vi "LVDimInterface.dic_command_service_local.vi"(1 "commandID":i32, 3 "data":string, 5 "error in (no error)":errorcluster) -> (15 "success":i32, 19 "error out":errorcluster)   [LabVIEW 2015, in "LVDimInterface.lvlib"]
doc: "This routine requests the execution of a command on the local (THIS) server, address and size contain the command parameters.\n\nThis routine allows clients (user interfaces for ex.) to send commands to be executed by internal servers.\n\nHistory: 16-DEC-2005, Dietrich Beck\n\nCopyright (C)\nGesellschaft für Schwerionenforschung, GSI\nPlanckstr. 1\n64291 Darmstadt\nGermany\n\nContact: D.Beck@gsi.de \n\nThis program is free software; you can redistribute it and/or modify it under the terms of the \nGNU General Public License as published by the Free Software Foundation; either version 2 of the license, or (at your option) any later version.\n\nThis program is distributed in the hope that it will be useful, but WITHOUT ANY WARRANTY; without even the implied warranty of MERCHANTABILITY or FITNESS FOR A PARTICULAR PURPOSE. See the GNU General License for more details (http://www.gnu.org).\n\nGesellschaft für Schwerionenforschung, GSI\nPlanckstr. 1, 64291 Darmstadt, Germany\nFor all questions and ideas contact D. Beck.\nLast update: 16-DEC-2005"
uses:
  LVDimInterface.lvlib
  LVDimInterface.queue type.ctl
  LVDimInterface.notifier type.ctl
panel:
  in  "notifierRef":T1
  in  "queueRef":T2
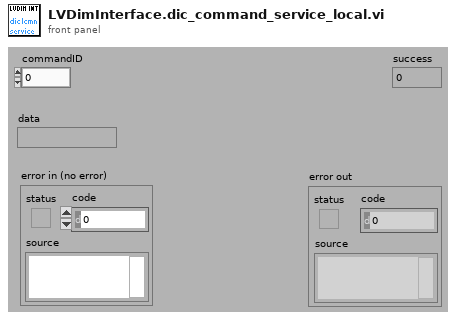
[diagram p1: front panel]
types:
  T1 = typedef "LVDimInterface.lvlib/LVDimInterface.notifier type.ctl" = refnum<notifier>
  T2 = typedef "LVDimInterface.lvlib/LVDimInterface.queue type.ctl" = refnum<queue>
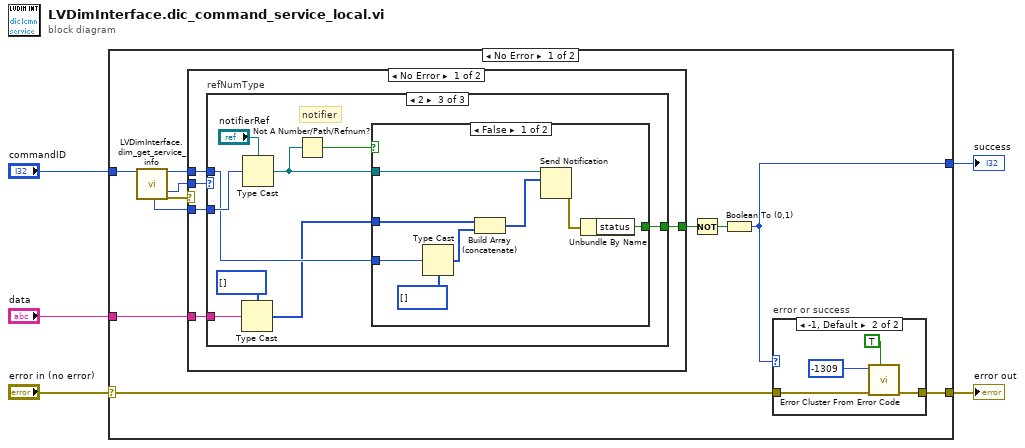
[diagram p0: block diagram]
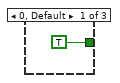
[diagram p2: hidden frame]
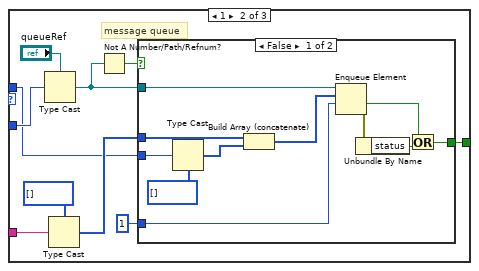
[diagram p3: hidden frame]
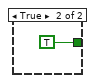
[diagram p4: hidden frame]
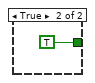
[diagram p5: hidden frame]
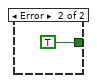
[diagram p6: hidden frame]
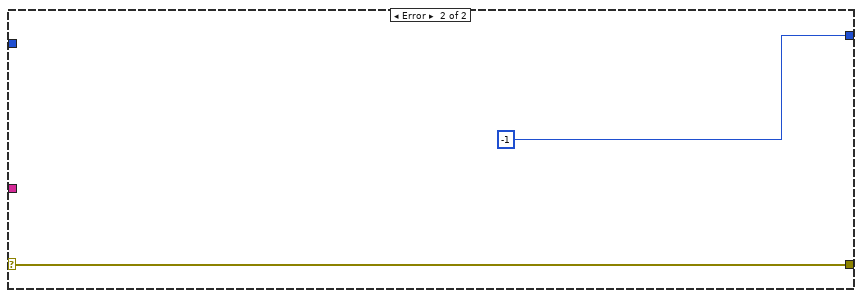
[diagram p8: hidden frame]
diagram:
  n1 = case shown="No Error" "error in (no error)" {
    selector: "error in (no error)" -> [w6 w69]
    tunnel: "commandID" -> [w15 _]
    tunnel: "data" -> [w12 _]
    tunnel: [w9 -1 ("success")] -> w4
    tunnel: [w16 w69] -> w3
    frame No Error {
      n2 = call "LVDimInterface.dim_get_service_info.vi"("callBackID"=w15) -> ("refNum"=w13:u32, "callBackID (out)"=w11:i32, "refNumType"=w14:i32, "error out"=w7:errorcluster)  [unwired: 9 in, 6 out]
      n3 = case shown="No Error" w7 {
        tunnel: w14 -> [w21 _]
        tunnel: w13 -> [w20 _]
        tunnel: w12 -> [w19 _]
        tunnel: w11 -> [w18 _]
        tunnel: [w17 TRUE ("status")] -> w10
        frame No Error {
          n4 = case "refNumType" shown="2" w21 {
            tunnel: w20 -> [_ w31 w53]
            tunnel: w19 -> [_ w27 w50]
            tunnel: w18 -> [_ w25 w47]
            tunnel: [TRUE ("status") w23 w45] -> w17
            frame 0, Default {
            }
            frame 1 {
              # "message queue"
              n5 = Type Cast(type="queueRef", x=w31) -> (*(type *) &x=w29:T2)
              n6 = Type Cast(type=i8[] [], x=w27) -> (*(type *) &x=w26:i8[])
              n7 = Not A Number/Path/Refnum?(number/path/refnum=w29) -> (NaN/Path/Refnum?=w32:bool)
              n8 = case shown="False" w32 {
                tunnel: w26 -> [w38 _]
                tunnel: 1 ("timeout") -> [w43 _]
                tunnel: [w33 TRUE] -> w23
                tunnel: w29 -> [w41 _]
                tunnel: w25 -> [w40 _]
                frame False {
                  n9 = Type Cast(type=i8[] [] ("element"), x=w40) -> (*(type *) &x=w37:i8[])
                  n10 = Build Array (concatenate)(w38, w37) -> (w36:i8[])
                  n11 = Enqueue Element(queue=w41, element=w36, timeout in ms (-1)=w43) -> (timed out?=w34:bool, error out=w42:errorcluster)  [unwired: 1 in, 1 out]
                  n12 = Unbundle By Name(w42) -> ("status"=w35:bool)
                  n13 = Or(x=w34, y=w35) -> (x .or. y?=w33:bool)
                }
                frame True {
                }
              }
            }
            frame 2 {
              # "notifier"
              n14 = Type Cast(type=i8[] [], x=w50) -> (*(type *) &x=w46:i8[])
              n15 = Type Cast(type="notifierRef", x=w53) -> (*(type *) &x=w49:T1)
              n16 = Not A Number/Path/Refnum?(number/path/refnum=w49) -> (NaN/Path/Refnum?=w48:bool)
              n17 = case shown="False" w48 {
                tunnel: w46 -> [w56 _]
                tunnel: [w61 TRUE ("status")] -> w45
                tunnel: w49 -> [w60 _]
                tunnel: w47 -> [w57 _]
                frame False {
                  n18 = Type Cast(type=i8[] [] ("element"), x=w57) -> (*(type *) &x=w55:i8[])
                  n19 = Build Array (concatenate)(w56, w55) -> (w54:i8[])
                  n20 = Send Notification(notification=w54, notifier=w60) -> (error out=w59:errorcluster)  [unwired: 1 in, 1 out]
                  n21 = Unbundle By Name(w59) -> ("status"=w61:bool)
                }
                frame True {
                }
              }
            }
          }
        }
        frame Error {
        }
      }
      n22 = Not(x=w10) -> (.not. x?=w8:bool)
      n23 = Boolean To (0,1)(Boolean=w8) -> (0, 1=w9:i16)
      n24 = case "error or success" shown="-1, Default" w9 {
        tunnel: w6 -> [w64 w67]
        tunnel: [w64 w68] -> w16
        frame 1 {
        }
        frame -1, Default {
          n25 = call <vilib>:"Error Cluster From Error Code.vi"("show call chain? (False)"=TRUE ("status"), "error in (no error)"=w67, "error code (0)"=-1309 ("code")) -> ("error out"=w68:errorcluster)  [unwired: 6 in]
        }
      }
    }
    frame Error {
    }
  }
  "success" <- w4
  "error out" <- w3
